vi "LER_ENET.vi"(3 "error in (no error)":errorcluster, 4 "Num de Bytes a Ser lido":u32=10, 5 "LNA VISA resource name":refnum<visa-resource-name>) -> (0 "error out":errorcluster, 1 "String Lida":string, 2 "VISA Out":refnum<visa-resource-name>)   [LabVIEW 2018]
panel:
  in  "Case Constant\n(See Context Help)":bool=TRUE
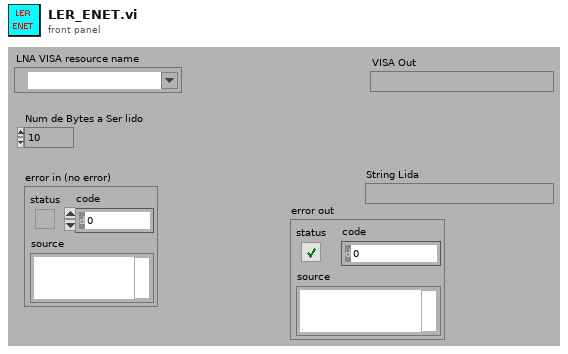
[diagram p1: front panel]
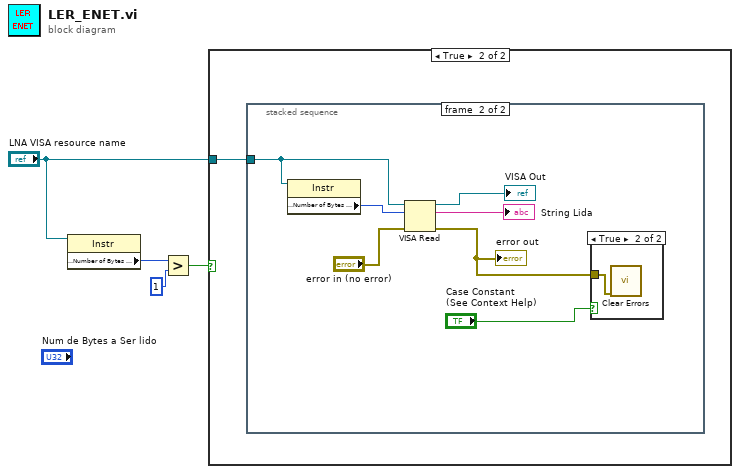
[diagram p0: block diagram]
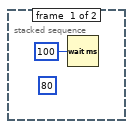
[diagram p3: hidden frame]
diagram:
  n1 = property class="Instr"(reference="LNA VISA resource name") -> ("Serial Settings:Number of Bytes at Serial Port"=w2:u32)  [unwired: 1 in, 2 out]
  n2 = Greater?(x=w2, y=u32 1) -> (0:w3:bool)
  n3 = case shown="True" w3 {
    tunnel: "LNA VISA resource name" -> [_ w5]
    frame False {
    }
    frame True {
      n4 = stacked-sequence {
        tunnel: w5 -> [_ w8]
        frame #0 {
          (unwired) u32 80 ("milliseconds to wait")
          n5 = Wait (ms)(milliseconds to wait=u32 100) -> ()  [unwired: 1 out]
        }
        frame #1 {
          n6 = property class="Instr"(reference=w8) -> ("Serial Settings:Number of Bytes at Serial Port"=w7:u32)  [unwired: 1 in, 2 out]
          n7 = VISA Read(VISA resource name=w8, byte count=w7, error in (no error)="error in (no error)") -> (VISA resource name out=→"VISA Out":refnum<visa-resource-name>, read buffer=→"String Lida":string, error out=w9:errorcluster)  [unwired: 1 out]
          "error out" <- w9
          n8 = case shown="True" "Case Constant\n(See Context Help)" {
            tunnel: w9 -> [_ w14]
            frame False {
            }
            frame True {
              n9 = call <vilib>:"Clear Errors.vi"("error in (no error)"=w14) -> ()  [unwired: 5 in, 2 out]
            }
          }
        }
      }
    }
  }
